vi "CreateFile.vi"(0 "object in":refnum<class "File.lvclass">, 5 "error in (no error)":errorcluster) -> (14 "object out":refnum<class "File.lvclass">, 19 "error out":errorcluster)   [LabVIEW 2021, in "File.lvclass"]
uses:
  File.lvclass
  File.lvclass/File.ctl
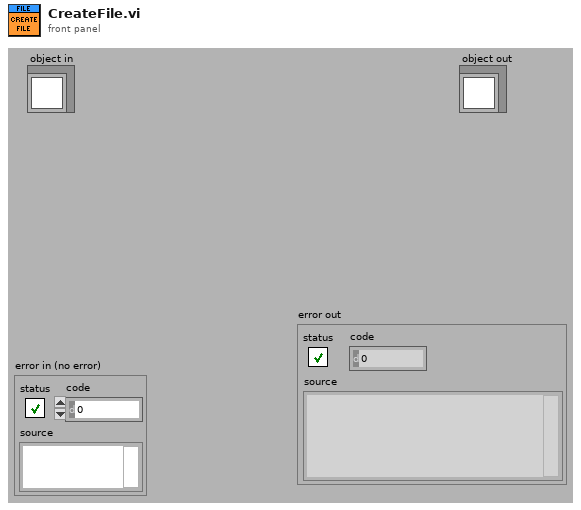
[diagram p1: front panel]
types:
  T1 = enum16{"open", "replace", "create", "open or create", "replace or create", "replace or create with confirmation"}
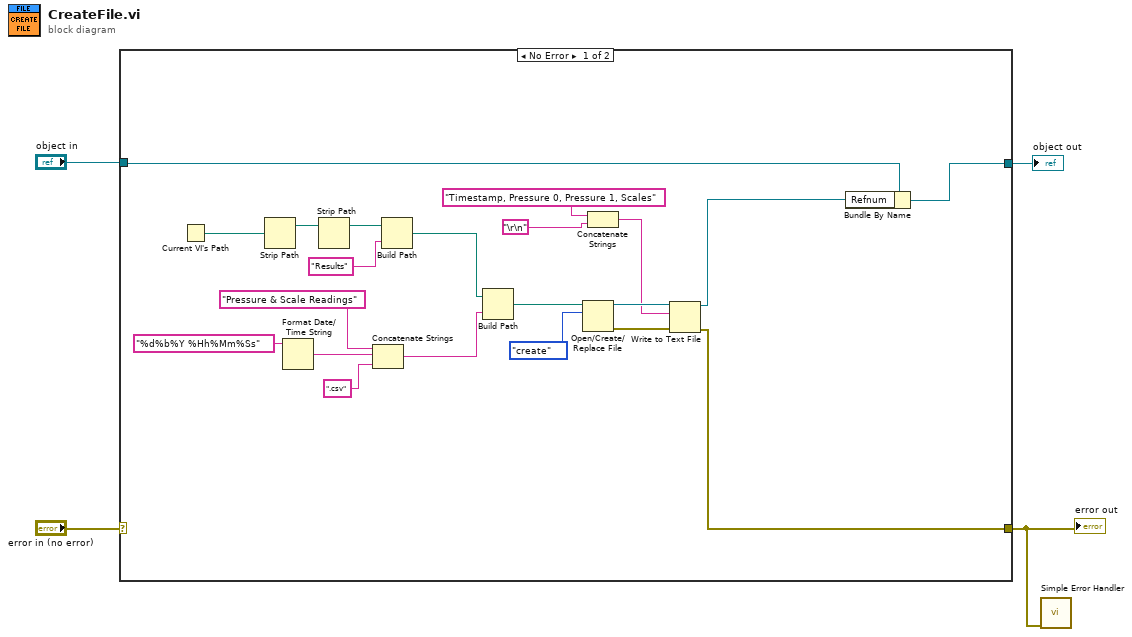
[diagram p0: block diagram]
diagram:
  n1 = case shown="No Error" "error in (no error)" {
    selector: "error in (no error)" -> [_ w27]
    tunnel: [w8 w27] -> w1
    tunnel: [w24 w26] -> w2
    tunnel: "object in" -> [w25 w26]
    frame No Error {
      n2 = Current VI's Path() -> (path=w19:path)
      n3 = Strip Path(path=w19) -> (stripped path=w6:path)  [unwired: 1 out]
      n4 = Format Date/Time String(time format string (%c)="%d%b%Y %Hh%Mm%Ss") -> (date/time string=w21:string)  [unwired: 2 in]
      n5 = Strip Path(path=w6) -> (stripped path=w5:path)  [unwired: 1 out]
      n6 = Concatenate Strings("Pressure & Scale Readings" ("string"), w21, ".csv" ("string")) -> (w16:string)
      n7 = Build Path(base path=w5, name or relative path="Results") -> (appended path=w17:path)
      n8 = Build Path(base path=w17, name or relative path=w16) -> (appended path=w10:path)
      n9 = Open/Create/Replace File(file path (use dialog)=w10, operation (0:open)=T1."create") -> (refnum out=w15:refnum<file>, error out=w11:errorcluster)  [unwired: 4 in, 1 out]
      n10 = Concatenate Strings("Timestamp, Pressure 0, Pressure 1, Scales", "\r\n") -> (w12:string)
      n11 = Write to Text File(file (use dialog)=w15, text=w12, error in=w11) -> (refnum out=w9:refnum<file>, error out=w8:errorcluster)  [unwired: 1 in, 1 out]
      n12 = Bundle By Name(cluster=w25, "Refnum"=w9) -> (w24:refnum<class "File.lvclass">)
    }
    frame Error {
    }
  }
  "error out" <- w1
  "object out" <- w2
  n13 = call <vilib>:"Simple Error Handler.vi"("error in (no error)"=w1) -> ()  [unwired: 4 in, 5 out]
